vi "Dresser DXD Revision Query.vi"(0 "VISA session":refnum<visa-resource-name>, 5 "Device Address (1)":T1=1 min=1 max=99 step=1, 11 "Error In (no error)":errorcluster) -> (4 "dup VISA session":refnum<visa-resource-name>, 6 "Returned String":string, 8 "Instr Driver Revision":string, 10 "Instr Firmware Revision":string, 15 "Error Out":errorcluster)   [LabVIEW 2015]
doc: "This VI queries the current Dresser DXD Series pressure transcducer firmware revision and instrument driver revision.\n\nThis Instrument Driver's Revision number is 2.0.0 and is known to be compatible with Instrument Firmware Revision 3.36\n\nDresser DXD Series Precision Digital Pressure Transducer LabVIEW Driver\nCreated By: BLOOMY CONTROLS, INC\n WINDSOR, CT 06095, USA\n 860-298-9925\n www.bloomy.com\nOriginal Release Date: February 11, 2000\nOriginally Developed in LabVIEW Version: 5.1\n\nModification History: \n(See the Read Me.txt file for specific changes and additions in each revision)\n\nV2.0.0 Mayl, 2002 LV 6.0.2"
uses:
  Type Defs/DXD Address.ctl
panel:
  # "For instructions on the use of this VI, press Ctrl+H to display the help window and move the mouse over the icon, controls, and indicators"
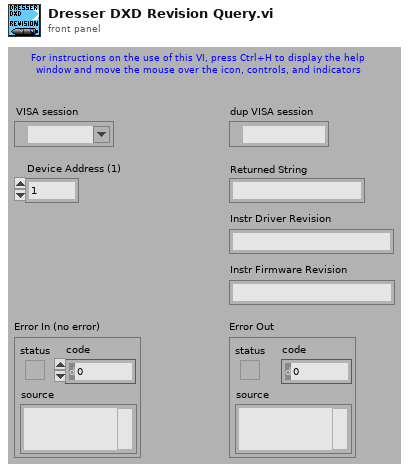
[diagram p1: front panel]
types:
  T1 = typedef "DXD Address.ctl" = i32
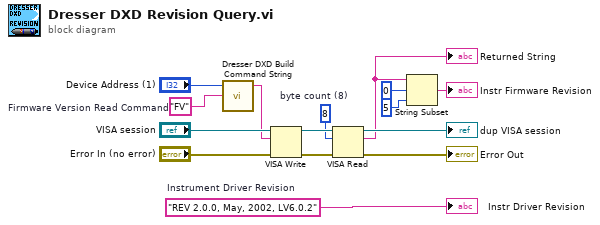
[diagram p0: block diagram]
diagram:
  w7 = u32 8  # byte count (8)
  w9 = "FV"  # Firmware Version Read Command
  w15 = "REV 2.0.0, May, 2002, LV6.0.2"  # Instrument Driver Revision
  n1 = call "Dresser DXD Build Command String.vi"("Command Mnemonic (\"\")"=w9, "DXD Address (1)"="Device Address (1)") -> ("Command String"=w8:string)  [unwired: 3 in]
  n2 = VISA Write(VISA resource name="VISA session", write buffer=w8, error in (no error)="Error In (no error)") -> (VISA resource name out=w12:refnum<visa-resource-name>, error out=w11:errorcluster)  [unwired: 1 out]
  n3 = VISA Read(VISA resource name=w12, byte count=w7, error in (no error)=w11) -> (VISA resource name out=→"dup VISA session":refnum<visa-resource-name>, read buffer=w1:string, error out=→"Error Out":errorcluster)  [unwired: 1 out]
  "Returned String" <- w1
  n4 = String Subset(string=w1, offset (0)=0, length (rest)=5 ("length (rest)")) -> (substring=→"Instr Firmware Revision":string)
  "Instr Driver Revision" <- w15
